vi "GetText.vi"(8 "error in":errorcluster, 11 "cRIO in":refnum<class "cfg cRIO root.lvclass">) -> (0 "error out":errorcluster, 1 "additional text":string, 2 "text":string, 3 "cRIO out":refnum<class "cfg cRIO root.lvclass">, 4 "glyph":string)   [LabVIEW 2013, in "cfg cRIO root.lvclass"]
uses:
  cfg cRIO root.lvclass
  cfg cRIO root.lvclass/cfg cRIO root.ctl
  criocfg/crio configuration.lvclass/crio configuration.ctl
  criocfg/crio configuration.lvclass
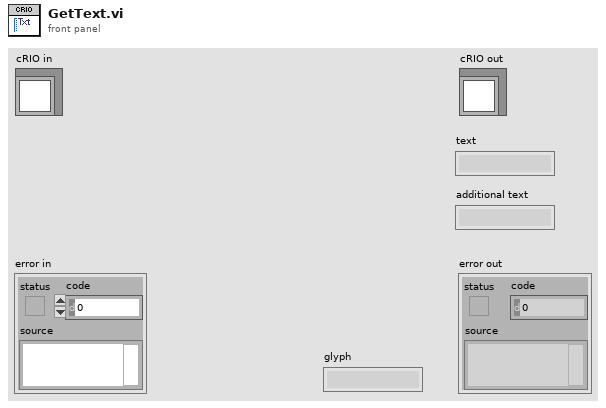
[diagram p1: front panel]
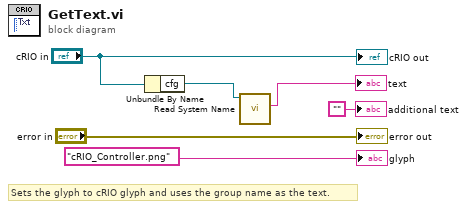
[diagram p0: block diagram]
diagram:
  # "Sets the glyph to cRIO glyph and uses the group name as the text."
  n1 = Unbundle By Name("cRIO in") -> ("cfg"=w2:refnum<class "crio configuration.lvclass">)
  n2 = call "Read System Name.vi"("crio configuration in"=w2) -> ("System Name"=→"text":string)  [unwired: 8 in, 2 out]
  "error out" <- "error in"
  "cRIO out" <- "cRIO in"
  "additional text" <- ""
  "glyph" <- "cRIO_Controller.png" ("glyph")
